vi "Act_BaseDatos_IV.vi"() -> ()   [LabVIEW 2020]
uses:
  <vilib>/httpClient/LabVIEWHTTPClient.lvlib
panel:
  out "Led Rele":bool
  out "Feedback [mA]":dbl
  out "Hora 2":string
  out "Hora":string
  out "Data":string
  in  "stop":bool
  out "error GET":errorcluster
  out "body GET":string
  out "headers GET":string
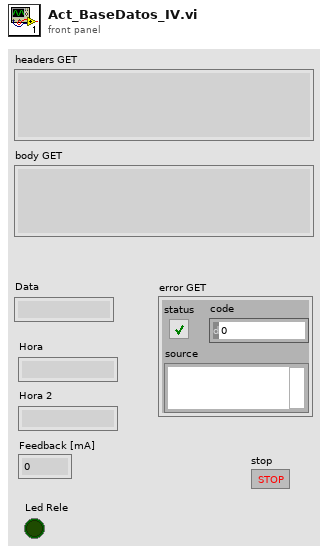
[diagram p1: front panel]
types:
  T1 = cluster{"Accionamiento":dbl, "Data":string, "Hora":string, "Led":bool}
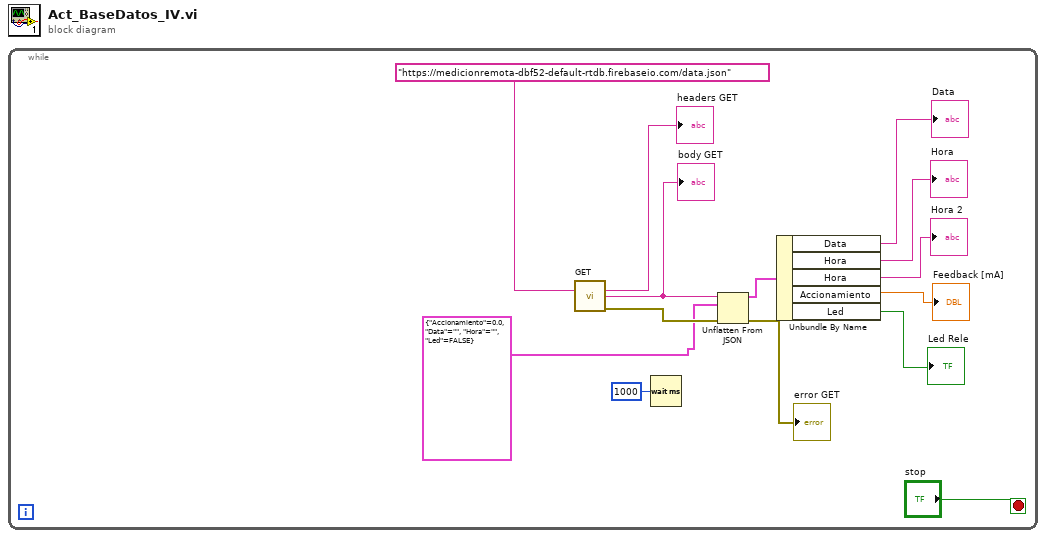
[diagram p0: block diagram]
diagram:
  n1 = while {
    stop <- "stop" stop-if-true
    n2 = call <vilib>:"GET.vi"("url"="https://medicionremota-dbf52-default-rtdb.firebaseio.com/data.json") -> ("headers"=→"headers GET":string, "body"=w11:string, "error out"=w10:errorcluster)  [unwired: 11 in, 1 out]
    "body GET" <- w11
    n3 = Wait (ms)(milliseconds to wait=u32 1000) -> ()  [unwired: 1 out]
    n4 = Unflatten From JSON(JSON string=w11, type and defaults=T1 {"Accionamiento"=0.0, "Data"="", "Hora"="", "Led"=FALSE}, error in (no error)=w10) -> (value=w1:T1, error out=→"error GET":errorcluster)  [unwired: 4 in]
    n5 = Unbundle By Name(w1) -> ("Data"=→"Data":string, "Hora"=→"Hora":string, "Hora"=→"Hora 2":string, "Accionamiento"=→"Feedback [mA]":dbl, "Led"=→"Led Rele":bool)
  }
